vi "startDriveMode.vi"(8 "error in (no error)":errorcluster, 9 "MotorController in":refnum<class "MotorController.lvclass">, 11 "interface object in":refnum<k20>) -> (0 "error out":errorcluster, 1 "MotorController out":refnum<class "MotorController.lvclass">, 2 "startDriveRes":u32, 3 "interface object out":refnum<k20>)   [LabVIEW 2018, in "MotorController.lvclass"]
uses:
  MotorController.lvclass
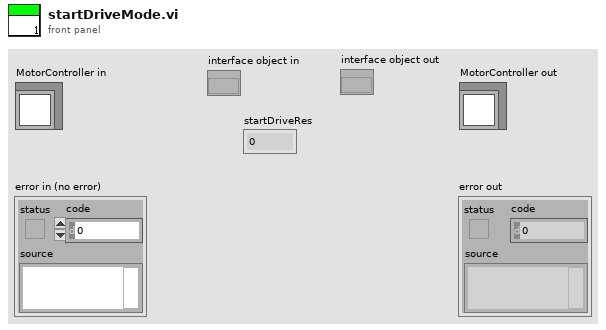
[diagram p1: front panel]
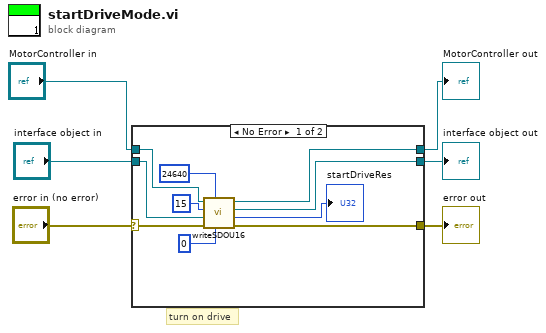
[diagram p0: block diagram]
diagram:
  # "turn on drive"
  n1 = case shown="No Error" "error in (no error)" {
    selector: "error in (no error)" -> [w15 w19]
    tunnel: [w7 w19] -> w5
    tunnel: [w9 w18] -> w3
    tunnel: "MotorController in" -> [w16 w18]
    tunnel: "interface object in" -> [w11 w17]
    tunnel: [w10 w17] -> w1
    frame No Error {
      n2 = call "writeSDOU16.vi"("object sub-index (0)"=u8 0, "object index"=u16 24640, "error in (no error)"=w15, "interface object in"=w11, "inputNumber"=u16 15, "MotorController in"=w16) -> ("error out"=w7:errorcluster, "completion code"=→"startDriveRes":u32, "interface object out"=w10:refnum<k20>, "MotorController out"=w9:refnum<class "MotorController.lvclass">)  [unwired: 2 in]
    }
    frame Error {
    }
  }
  "error out" <- w5
  "MotorController out" <- w3
  "interface object out" <- w1
